vi "get waveform - 8bit.vi"(8 "error in (no error)":errorcluster caption="에러 입력(에러 없음)", 11 "Waveform Obj 입력":refnum<class "Waveform Obj.lvclass">) -> (0 "error out":errorcluster caption="에러 출력", 1 "8bit memory data":u8[](array[numeric]), 2 "8bit waveform":waveform(i8), 3 "Waveform Obj 출력":refnum<class "Waveform Obj.lvclass">)   [LabVIEW 2020, in "Waveform Obj.lvclass"]
uses:
  Waveform Obj.lvclass
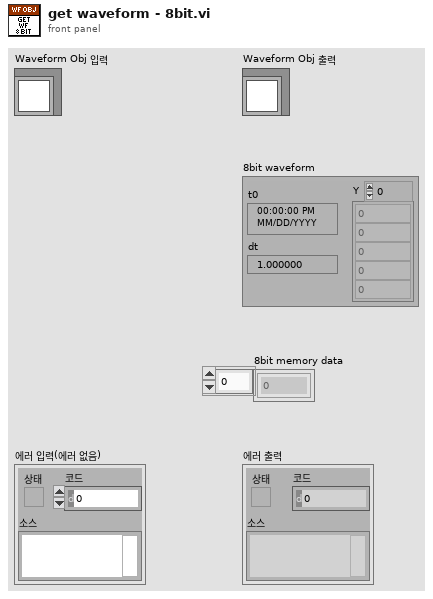
[diagram p1: front panel]
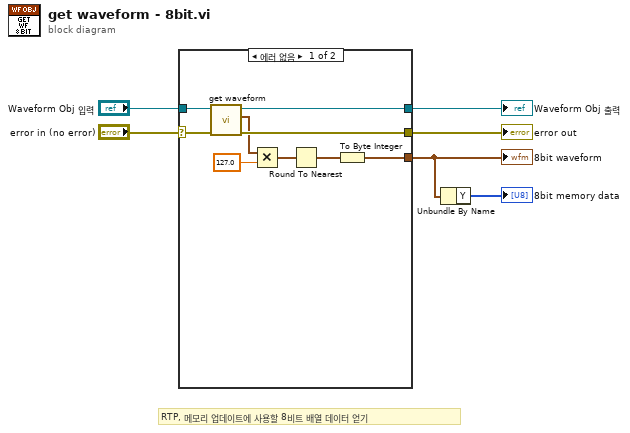
[diagram p0: block diagram]
diagram:
  # "RTP, 메모리 업데이트에 사용할 8비트 배열 데이터 얻기"
  n1 = case shown="에러 없음" "error in (no error)" {
    selector: "error in (no error)" -> [w15 w17]
    tunnel: [w14 w17] -> w5
    tunnel: [w12 w16] -> w3
    tunnel: "Waveform Obj 입력" -> [w13 w16]
    tunnel: [w7 _] -> w2
    frame No Error {
      n2 = call-dynamic "get waveform.vi"("error in (no error)"=w15, "Waveform Obj 입력"=w13) -> ("error out"=w14:errorcluster, "waveform"=w11:waveform(dbl), "Waveform Obj 출력"=w12:refnum<class "Waveform Obj.lvclass">)  [unwired: 7 in]
      n3 = Multiply(x=w11, y=127.0) -> (x*y=w9:waveform(dbl))
      n4 = Round To Nearest(number=w9) -> (nearest integer value=w8:waveform(dbl))
      n5 = To Byte Integer(number=w8) -> (8bit integer=w7:waveform(i8))
    }
    frame Error {
    }
  }
  "error out" <- w5
  "Waveform Obj 출력" <- w3
  "8bit waveform" <- w2
  n6 = Unbundle By Name(w2) -> ("Y"=→"8bit memory data":i8[])
